vi "IntersectPoint.vi"(8 "Max Dist":dbl=40.0, 10 "Against Array":cluster{"X":dbl, "Y":dbl, "Z":dbl}[](array[cluster]), 11 "Test Array":cluster{"X":dbl, "Y":dbl, "Z":dbl}[](array[cluster])) -> (0 "Intersect Point":cluster{"X":dbl, "Y":dbl, "Z":dbl}, 1 "Distance":dbl, 2 "With Line?":bool=TRUE, 3 "Check":bool)   [LabVIEW 2014]
panel:
  in  "milliseconds to wait":u32
  out "Towards?":bool
  out "ub Range?":bool
  out "ua Range?":bool
  out "iy":dbl
  out "ix":dbl
  out "ub":dbl
  out "ua":dbl
  out "XY Graph":cluster{dbl[], dbl[]}[](graph)=[{[1.0, 2.0], [1.0, 3.0]}, {[3.0, 4.0], [4.0, 6.0]}]
  # "Posit"
  # "2nd"
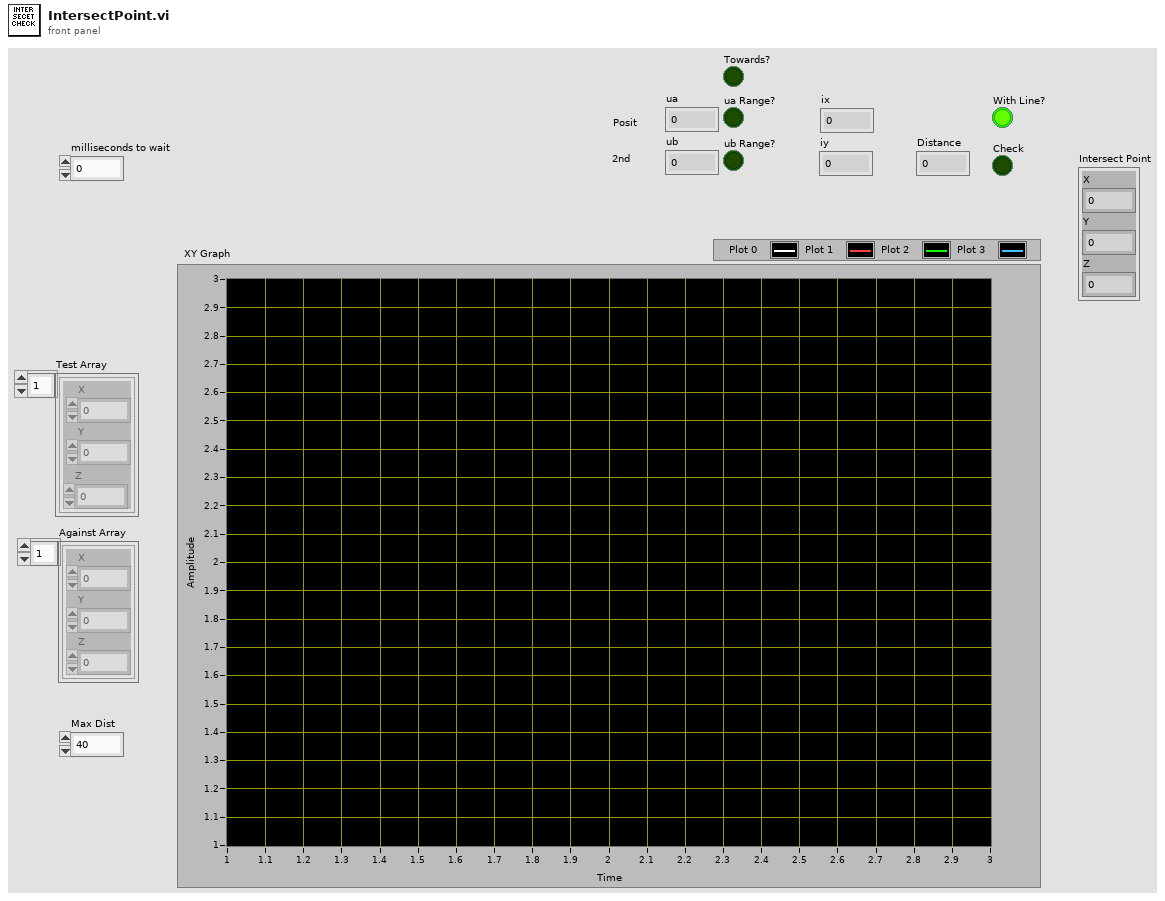
[diagram p1: front panel]
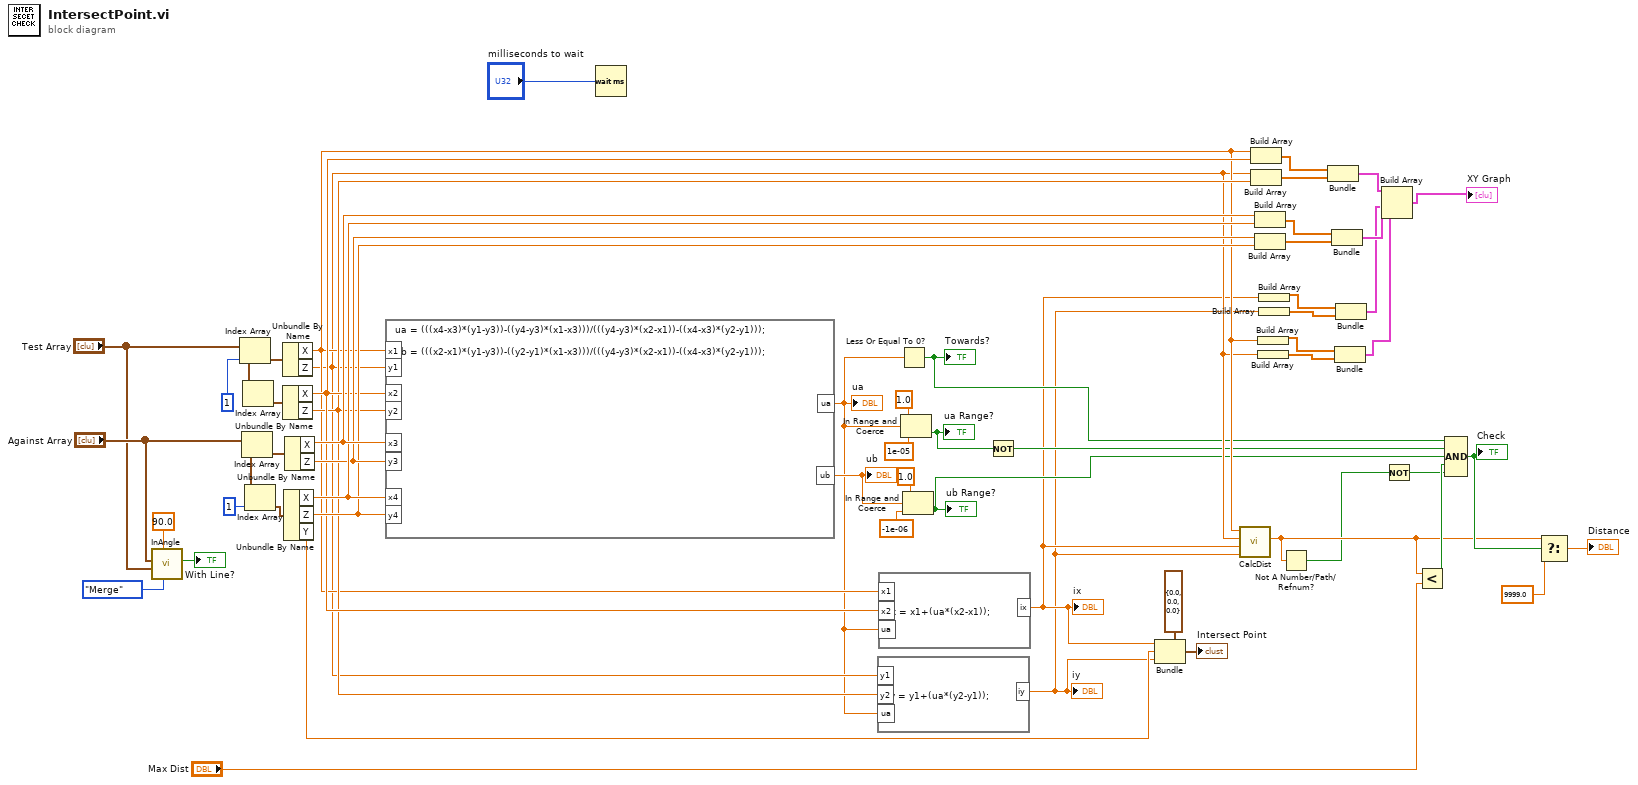
[diagram p0: block diagram]
diagram:
  n1 = call "InAngle.vi"("Function"=enum16{"Posit", "Merge"}."Merge", "Angle"=90.0, "2nd Array (Start)"="Test Array", "Base Array (End)"="Against Array") -> ("In Angle?"=→"With Line?":bool)  [unwired: 7 in]
  n2 = Index Array(array="Test Array", index=1) -> (element=w36:cluster{"X":dbl, "Y":dbl, "Z":dbl})
  n3 = Index Array(array="Against Array") -> (element=w53:cluster{"X":dbl, "Y":dbl, "Z":dbl})  [unwired: 1 in]
  n4 = Index Array(array="Test Array") -> (element=w37:cluster{"X":dbl, "Y":dbl, "Z":dbl})  [unwired: 1 in]
  n5 = Index Array(array="Against Array", index=1) -> (element=w54:cluster{"X":dbl, "Y":dbl, "Z":dbl})
  n6 = Unbundle By Name(w36) -> ("X"=w32:dbl, "Z"=w31:dbl)
  n7 = Unbundle By Name(w37) -> ("X"=w42:dbl, "Z"=w41:dbl)
  n8 = Unbundle By Name(w54) -> ("X"=w45:dbl, "Z"=w43:dbl, "Y"=w15:dbl)
  n9 = Unbundle By Name(w53) -> ("X"=w46:dbl, "Z"=w44:dbl)
  n10 = formula code="ua = (((x4-x3)*(y1-y3))-((y4-y3)*(x1-x3)))/(((y4-y3)*(x2-x1))-((x4-x3)*(y2-y1)));\n\nub = (((x2-x1)*(y1-y3))-((y2-y1)*(x1-x3)))/(((y4-y3)*(x2-x1))-((x4-x3)*(y2-y1)));"("x1"=w32, "x2"=w42, "y1"=w31, "y2"=w41, "x3"=w46, "y3"=w44, "x4"=w45, "y4"=w43) -> ("ua"=w25:dbl, "ub"=w28:dbl)
  "ua" <- w25
  "ub" <- w28
  n11 = Wait (ms)(milliseconds to wait="milliseconds to wait") -> ()  [unwired: 1 out]
  n12 = formula code="iy = y1+(ua*(y2-y1));"("y1"=w31, "y2"=w41, "ua"=w25) -> ("iy"=w13:dbl)
  "iy" <- w13
  n13 = formula code="ix = x1+(ua*(x2-x1));"("x1"=w32, "x2"=w42, "ua"=w25) -> ("ix"=w16:dbl)
  "ix" <- w16
  n14 = Less Or Equal To 0?(x=w25) -> (x <= 0?=w23:bool)
  "Towards?" <- w23
  n15 = In Range and Coerce(upper limit=1.0, x=w25, lower limit=1e-05) -> (In Range?=w24:bool)  [unwired: 1 out]
  "ua Range?" <- w24
  n16 = In Range and Coerce(upper limit=1.0, x=w28, lower limit=-1e-06) -> (In Range?=w21:bool)  [unwired: 1 out]
  "ub Range?" <- w21
  n17 = Not(x=w24) -> (.not. x?=w22:bool)
  n18 = Bundle(cluster=cluster{"X":dbl, "Y":dbl, "Z":dbl} {"X"=0.0, "Y"=0.0, "Z"=0.0} ("Map data"), "X"=w16, "Y"=w15, "Z"=w13) -> (→"Intersect Point":cluster{"X":dbl, "Y":dbl, "Z":dbl})
  n19 = call "CalcDist.vi"("Y2"=w13, "X2"=w16, "Y1"=w31, "X1"=w32) -> ("Distance"=w10:dbl)  [unwired: 7 in]
  n20 = Build Array(w32, w42) -> (w52:dbl[])
  n21 = Build Array(w31, w41) -> (w51:dbl[])
  n22 = Build Array(w46, w45) -> (w48:dbl[])
  n23 = Build Array(w44, w43) -> (w49:dbl[])
  n24 = Build Array(w32) -> (w34:dbl[])
  n25 = Build Array(w31) -> (w35:dbl[])
  n26 = Build Array(w16) -> (w40:dbl[])
  n27 = Build Array(w13) -> (w39:dbl[])
  n28 = Not A Number/Path/Refnum?(number/path/refnum=w10) -> (NaN/Path/Refnum?=w6:bool)
  n29 = Bundle(w52, w51) -> (w50:cluster{dbl[], dbl[]})  [unwired: 1 in]
  n30 = Bundle(w48, w49) -> (w47:cluster{dbl[], dbl[]})  [unwired: 1 in]
  n31 = Bundle(w34, w35) -> (w33:cluster{dbl[], dbl[]})  [unwired: 1 in]
  n32 = Bundle(w40, w39) -> (w38:cluster{dbl[], dbl[]})  [unwired: 1 in]
  n33 = Build Array(w50, w47, w38, w33) -> (→"XY Graph":cluster{dbl[], dbl[]}[])
  n34 = Not(x=w6) -> (.not. x?=w12:bool)
  n35 = Less?(x=w10, y="Max Dist") -> (x < y?=w19:bool)
  n36 = Compound Arithmetic op=AND(w23, w22, w21, w19, w12) -> (w11:bool)
  "Check" <- w11
  n37 = Select(t=w10, s=w11, f=9999.0 ("t")) -> (s? t:f=→"Distance":dbl)
